vi "Analog Input Read.vi"(8 "error in (no error)":errorcluster, 11 "Analog Input in":refnum<class "NI Analog Input.lvclass">) -> (0 "error out":errorcluster, 2 "data":dbl[][](array[numeric]) format="%0.2f", 3 "Analog Input out":refnum<class "NI Analog Input.lvclass">)   [LabVIEW 2023, in "HardwareAbstractionLayer_LVOOP.lvlib" / "NI Analog Input.lvclass"]
uses:
  NI Analog Input.lvclass
  NI Analog Input.lvclass/NI Analog Input.ctl
  <vilib>/DAQmx/read.llb/DAQmx Read (Analog 2D DBL NChan NSamp).vi
  <vilib>/DAQmx/miscellaneous.llb/DAQmx Fill In Error Info.vi
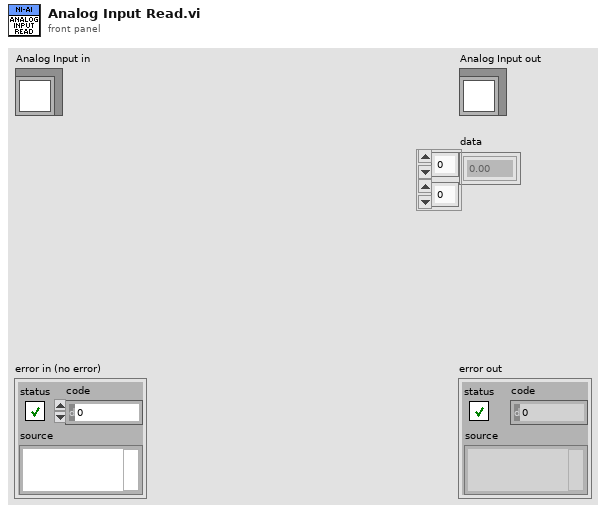
[diagram p1: front panel]
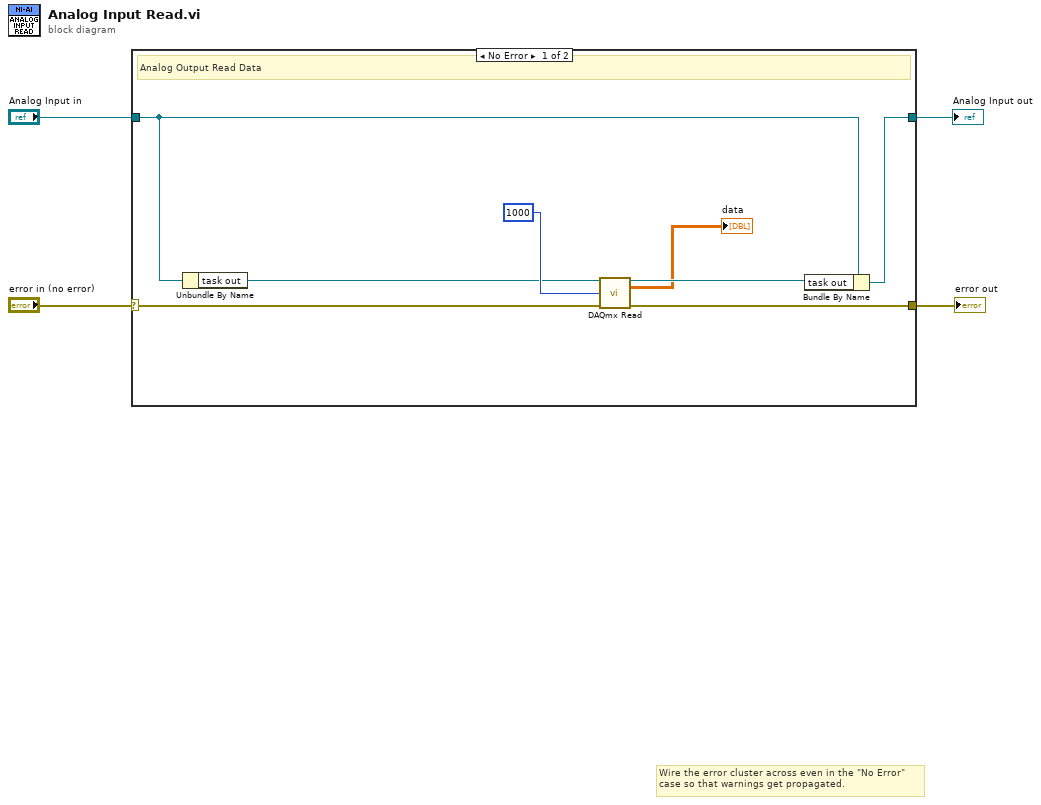
[diagram p0: block diagram]
diagram:
  # "Wire the error cluster across even in the \"No Error\"\ncase so that warnings get propagated."
  n1 = case shown="No Error" "error in (no error)" {
    selector: "error in (no error)" -> [w5 w14]
    tunnel: [w12 w14] -> w3
    tunnel: [w10 w13] -> w1
    tunnel: "Analog Input in" -> [w11 w13]
    frame No Error {
      # "Analog Output Read Data"
      n2 = Unbundle By Name(w11) -> ("task out"=w6:refnum<k21>)
      n3 = call-poly <vilib>:"DAQmx Read.vi"("task/channels in"=w6, "number of samples per channel"=1000, "error in"=w5) -> ("task out"=w9:refnum<k21>, "data"=→"data":dbl[][], "error out"=w12:errorcluster)  [unwired: 10 in]
      n4 = Bundle By Name(cluster=w11, "task out"=w9) -> (w10:refnum<class "NI Analog Input.lvclass">)
    }
    frame Error {
    }
  }
  "error out" <- w3
  "Analog Input out" <- w1
